vi "Get Application Name.vi"(8 "error in (no error)":errorcluster) -> (0 "error out":errorcluster, 3 "Application Name":string)   [LabVIEW 2016, in "System.lvlib"]
uses:
  System.lvlib
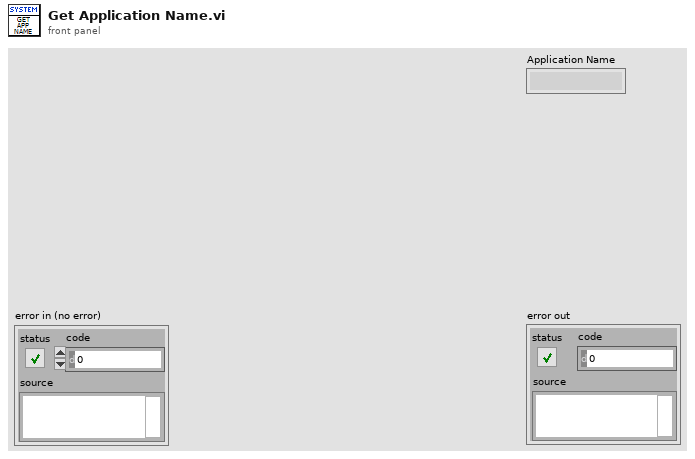
[diagram p1: front panel]
types:
  T1 = typedef "System.lvlib/Control_Variant Data Reference.ctl" = refnum<data-value>
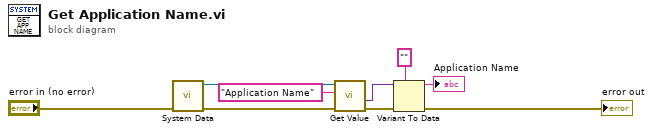
[diagram p0: block diagram]
diagram:
  n1 = call "System Data.vi"("error in (no error)"="error in (no error)") -> ("error out"=w8:errorcluster, "System Data Reference"=w9:T1)  [unwired: 9 in]
  n2 = call "Get Value.vi"("error in (no error)"=w8, "Name"="Application Name", "Data Reference"=w9) -> ("error out"=w6:errorcluster, "Value"=w5:variant)  [unwired: 7 in]
  n3 = Variant To Data(error in=w6, type="", Variant=w5) -> (data=→"Application Name":string, error out=→"error out":errorcluster)
